vi "_092.vi"() -> ()   [LabVIEW 2020]
panel:
  out "String 3":string
  out "String 2":string
  out "Numeric 6":dbl
  out "String":string
  in  "Numeric 5":dbl
  out "Boolean":bool
  out "Numeric 4":dbl
  out "Numeric 3":dbl
  out "Numeric 2":dbl
  in  "Numeric":dbl
  # "Control wired to another Control :"
  # "Mismatch Datatypes :"
  # "Indicator wired to another indicator :"
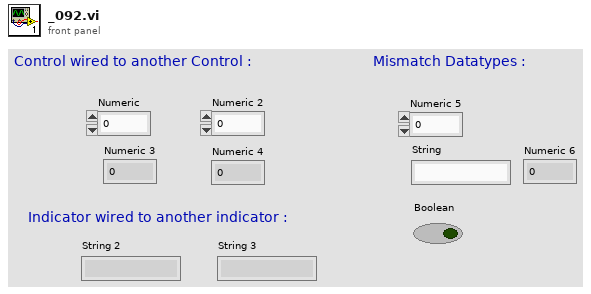
[diagram p1: front panel]
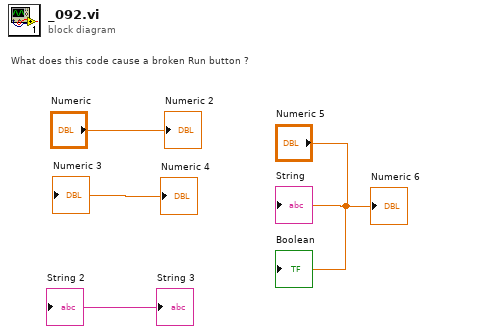
[diagram p0: block diagram]
diagram:
  # "What does this code cause a broken Run button ?"
  "Numeric 2" <- "Numeric"
  "Numeric 3" <- "Numeric 4"
  "Boolean" <- "Numeric 5"
  "String" <- "Numeric 5"
  "Numeric 6" <- "Numeric 5"
  "String 2" <- "String 3"
